vi "Init.vi"(8 "error in (no error)":errorcluster, 11 "RealSubject1 in":refnum<class "RealSubject1.lvclass">) -> (0 "error out":errorcluster, 3 "RealSubject1 out":refnum<class "RealSubject1.lvclass">)   [LabVIEW 2014, in "Normal Proxy.lvlib" / "RealSubject1.lvclass"]
uses:
  RealSubject1.lvclass
  Subject/Subject.lvclass/Subject.ctl
  Subject/Subject.lvclass
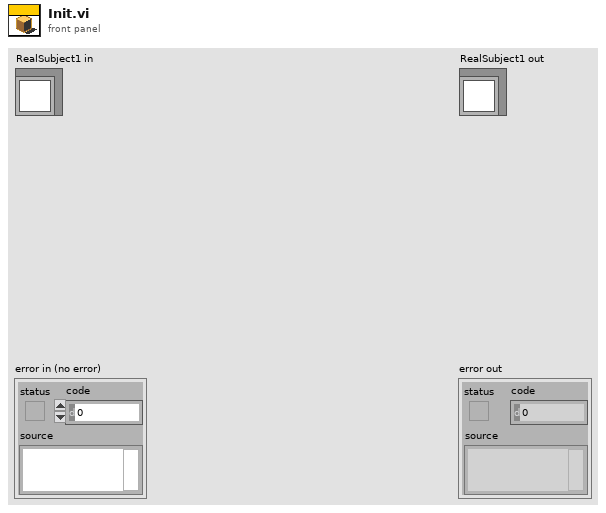
[diagram p1: front panel]
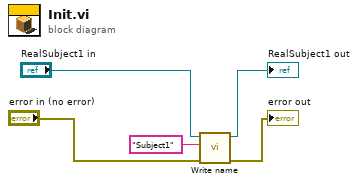
[diagram p0: block diagram]
diagram:
  n1 = call "Write name.vi"("error in (no error)"="error in (no error)", "name"="Subject1", "Subject in"="RealSubject1 in") -> ("error out"=→"error out":errorcluster, "Subject out"=→"RealSubject1 out":refnum<class "RealSubject1.lvclass">)  [unwired: 7 in]
